vi "ZDataVis_sliceTest.vi"(10 "Vsd DVR":refnum<data-value>, 11 "I DVR":refnum<data-value>) -> ()   [LabVIEW 2016]
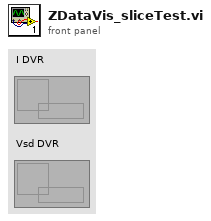
[diagram p1: front panel]
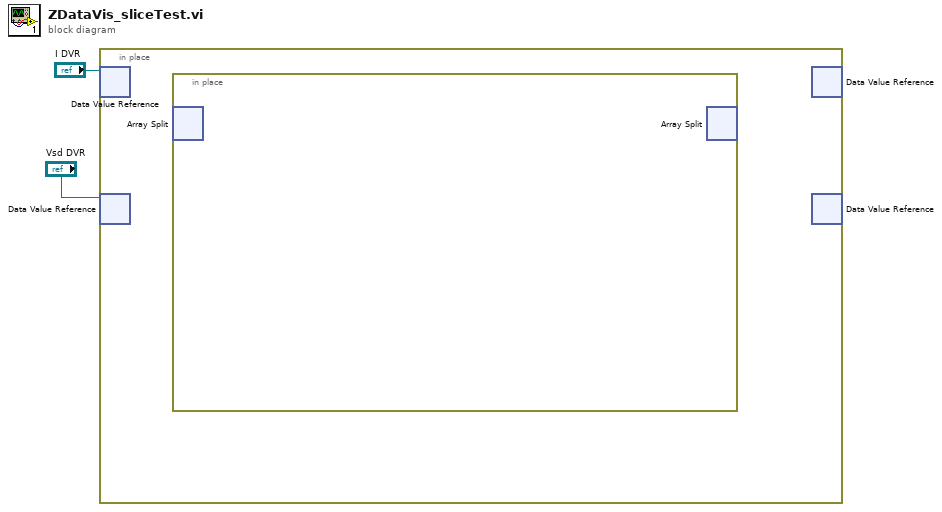
[diagram p0: block diagram]
diagram:
  n1 = in-place {
    n2 = in-place-dvr #1("I DVR") -> ()  [unwired: 2 out]
    n3 = in-place-dvr #2("Vsd DVR") -> ()  [unwired: 2 out]
    n4 = in-place {
      n5 = in-place-split #3() -> ()  [unwired: 2 in, 2 out]
      n6 = in-place-split #3() -> ()  [unwired: 2 in, 2 out]
    }
    n7 = in-place-dvr #1() -> ()  [unwired: 1 in, 2 out]
    n8 = in-place-dvr #2() -> ()  [unwired: 1 in, 2 out]
  }
